vi "SaveFileOnMP.vi"(8 "error in":errorcluster, 9 "FileName":string, 10 "Code sent":string, 11 "VISA in":refnum<visa-resource-name>) -> (0 "error out":errorcluster, 2 "Visible":bool, 3 "VISA out":refnum<visa-resource-name>)   [LabVIEW 2016]
panel:
  out "VISA in 2":refnum<visa-resource-name>
  out "Code read":string
  out "message":string
  in  "Done":bool
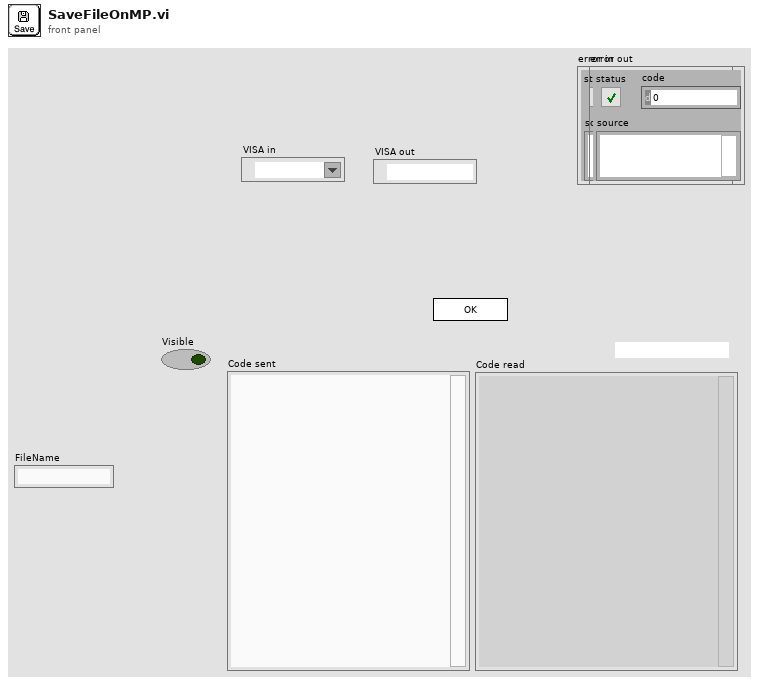
[diagram p1: front panel]
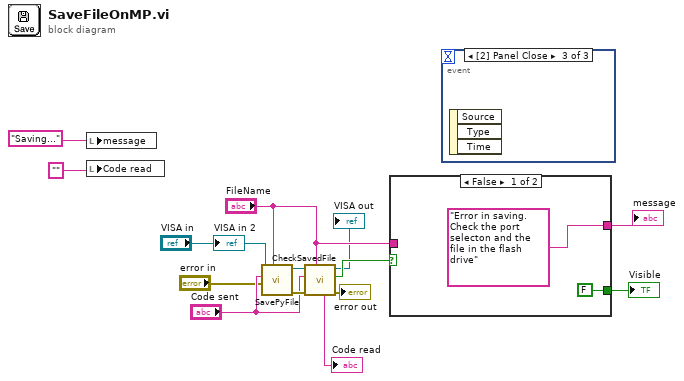
[diagram p0: block diagram]
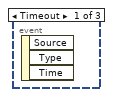
[diagram p2: hidden frame]
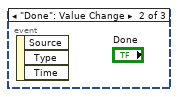
[diagram p3: hidden frame]
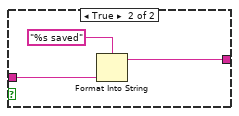
[diagram p4: hidden frame]
diagram:
  n1 = local write "message"("Saving..." ("Code read")) -> ()
  n2 = local write "Code read"("" ("Code read")) -> ()
  n3 = call "SavePyFile.vi"("Name"="FileName", "error in"="error in", "Python Code"="Code sent", "VISA in"="VISA in") -> ("error out"=w11:errorcluster, "VISA out"=w12:refnum<visa-resource-name>)  [unwired: 5 in, 1 out]
  n4 = call "CheckSavedFile.vi"("Name"="FileName", "error in (no error)"=w11, "All Code"="Code sent", "VISA in"=w12) -> ("error out"=→"error out":errorcluster, "Success?"=w13:bool, "VISA out"=→"VISA out":refnum<visa-resource-name>, "Saved Contents"=→"Code read":string)  [unwired: 3 in, 1 out]
  n5 = case shown="False" w13 {
    tunnel: "FileName" -> [_ w18]
    tunnel: [FALSE ("Visible") _] -> w14
    tunnel: ["Error in saving. Check the port selecton and the file in the flash drive" ("message") w17] -> w9
    frame False {
    }
    frame True {
      n6 = Format Into String(format string="%s saved" ("message"), w18) -> (resulting string=w17:string)  [unwired: 2 in, 1 out]
    }
  }
  "Visible" <- w14
  "message" <- w9
  n7 = event shown="[2] Panel Close" {
    selector: _ -> [_ _ _]
    dyn-events: _ -> [_ _ _]
    timeout: _ -> [_ _ _]
    event Timeout {
      n8 = event-data() -> ()  [unwired: 1 in, 3 out]
    }
    event "Done": Value Change {
      n9 = event-data() -> ()  [unwired: 1 in, 3 out]
    }
    event Panel Close {
      n10 = event-data() -> ()  [unwired: 1 in, 3 out]
    }
  }
  "VISA in 2" <- "VISA in"
